vi "DDS Read Register.vi"(6 "channel number (1)":u8=1 min=1 max=4 step=1, 8 "error in (no error)":errorcluster, 9 "# RAM words (0)":i32, 10 "Register":T3, 11 "DDS ref in":T1={"NI USB-8451 device reference"="", "DIO port"=0, "Serial Clock Rate [kHz]"=1000}) -> (0 "error out":errorcluster, 2 "Read data":u8[](array[numeric]), 3 "DDS ref out":T1={"NI USB-8451 device reference"="", "DIO port"=0, "Serial Clock Rate [kHz]"=1000})   [LabVIEW 2013, in "DDS.lvlib"]
doc: "Reads the current value of the specified register in the specified channel. Note that only the profile register currently selected by the external profile pins can be read."
uses:
  DDS.lvlib
  Controls/AD9910 registers.ctl
  Controls/DDS Box Device Reference.ctl
  <vilib>/ni845x/ni845x.llb/ni845xControl.ctl
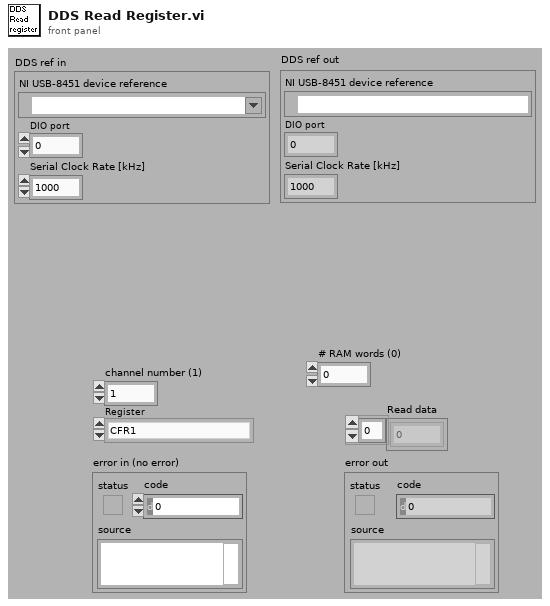
[diagram p1: front panel]
types:
  T1 = typedef "DDS.lvlib/DDS Box Device Reference.ctl" = cluster{"NI USB-8451 device reference":T2, "DIO port":u8, "Serial Clock Rate [kHz]":u16}
  T2 = typedef "ni845xControl.ctl" = refnum<k21>
  T3 = typedef "DDS.lvlib/AD9910 registers.ctl" = enum16{"CFR1", "CFR2", "CFR3", "Auxiliary DAC Control", "I/0 Update Rate", "Frequency Tuning Word", "Phase Offset Word", "Amplitude Scale Factor", "Multichip Sync", "Digital Ramp Limit", "Digital Ramp Step Size", "Digital Ramp Rate", "Single Tone Profile 0", "Single Tone Profile 1", "Single Tone Profile 2", "Single Tone Profile 3", "Single Tone Profile 4", "Single Tone Profile 5", "Single Tone Profile 6", "Single Tone Profile 7", "RAM Profile 0", "RAM Profile 1", "RAM Profile 2", "RAM Profile 3", "RAM Profile 4", "RAM Profile 5", "RAM Profile 6", "RAM Profile 7", "RAM"}
  T4 = typedef "ni845xSpiScriptControl.ctl" = refnum<k20>
  T5 = typedef "DDS.lvlib/DDS CS pins.ctl" = enum8{"IO reset", "Ch. 4 CS", "Ch. 3 CS", "Ch. 2 CS", "Ch. 1 CS"}
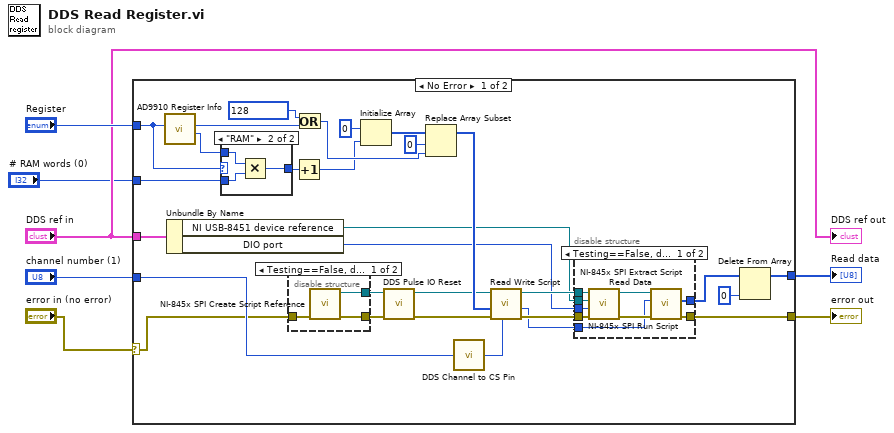
[diagram p0: block diagram]
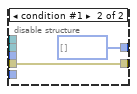
[diagram p3: hidden frame]
diagram:
  n1 = case shown="No Error" "error in (no error)" {
    selector: "error in (no error)" -> [w13 w56]
    tunnel: "DDS ref in" -> [w36 _]
    tunnel: "Register" -> [w12 _]
    tunnel: [w22 w56] -> w5
    tunnel: [w17 _] -> w4
    tunnel: "channel number (1)" -> [w15 _]
    tunnel: "# RAM words (0)" -> [w11 _]
    frame No Error {
      n2 = call "AD9910 Register Info.vi"("Register"=w12) -> ("Number of Bytes"=w10:i32, "Address"=w21:u8)  [unwired: 9 in]
      n3 = Unbundle By Name(w36) -> ("NI USB-8451 device reference"=w25:T2, "DIO port"=w24:u8)
      n4 = case shown="\"RAM\"" w12 {
        tunnel: w10 -> [w37 w39]
        tunnel: [w37 w38] -> w9
        tunnel: w11 -> [_ w40]
        frame "CFR1", Default {
        }
        frame "RAM" {
          n5 = Multiply(x=w39, y=w40) -> (x*y=w38:i32)
        }
      }
      n6 = disable-structure shown="Testing==False, default" {
        disable-tunnel: w13 -> [w54 w55]
        disable-tunnel: [w53 _] -> w35
        disable-tunnel: [w52 w55] -> w34
        frame condition #0 (active) {
          n7 = call <vilib>:"NI-845x SPI Create Script Reference.vi"("error in (no error)"=w54) -> ("error out"=w52:errorcluster, "spi script reference"=w53:T4)  [unwired: 9 in]
        }
        frame condition #1 {
        }
      }
      n8 = Increment(x=w9) -> (x+1=w8:i32)
      n9 = Or(x=u8 128, y=w21) -> (x .or. y?=w19:u8)
      n10 = Initialize Array(u8 0 ("element"), w8) -> (w32:u8[])
      n11 = call "DDS Pulse IO Reset.vi"("error in (no error)"=w34, "spi script reference in"=w35) -> ("error out"=w29:errorcluster, "spi script reference out"=w28:T4)  [unwired: 8 in]
      n12 = Replace Array Subset(array=w32, new element=w19, index=0) -> (w30:u8[])
      n13 = call "DDS Channel to CS Pin.vi"("channel number (1)"=w15) -> ("CS pin"=w14:T5)
      n14 = call "Read Write Script.vi"("chip select (0)"=w14, "error in (no error)"=w29, "Write Data"=w30, "spi script reference in"=w28) -> ("error out"=w27:errorcluster, "script read index"=w23:u32, "spi script reference out"=w26:T4)  [unwired: 5 in]
      n15 = disable-structure shown="Testing==False, default" {
        disable-tunnel: w27 -> [w49 w51]
        disable-tunnel: w26 -> [w48 _]
        disable-tunnel: w25 -> [w47 _]
        disable-tunnel: w24 -> [w46 _]
        disable-tunnel: w23 -> [w43 _]
        disable-tunnel: [w42 w51] -> w22
        disable-tunnel: [w41 u8[] [] ("read data")] -> w18
        frame condition #0 (active) {
          n16 = call <vilib>:"NI-845x SPI Run Script.vi"("error in (no error)"=w49, "port (0)"=w46, "device reference in"=w47, "spi script reference in"=w48) -> ("error out"=w45:errorcluster, "spi script reference out"=w44:T4)  [unwired: 5 in, 1 out]
          n17 = call <vilib>:"NI-845x SPI Extract Script Read Data.vi"("error in (no error)"=w45, "script read index"=w43, "spi script reference in"=w44) -> ("error out"=w42:errorcluster, "read data"=w41:u8[])  [unwired: 6 in, 1 out]
        }
        frame condition #1 {
        }
      }
      n18 = Delete From Array(array=w18, index=0) -> (array with subset deleted=w17:u8[])  [unwired: 1 in, 1 out]
    }
    frame Error {
    }
  }
  "error out" <- w5
  "Read data" <- w4
  "DDS ref out" <- "DDS ref in"
